vi "Create.vi"() -> (8 "Moving Ripple Noise":refnum<class "Moving Ripple Noise.lvclass">)   [LabVIEW 2020, in "Moving Ripple Noise.lvclass"]
uses:
  Moving Ripple Noise.lvclass
  Moving Ripple Noise.lvclass/Moving Ripple Noise.ctl
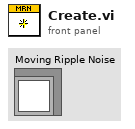
[diagram p1: front panel]
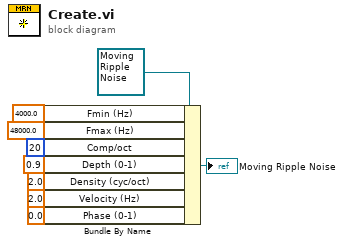
[diagram p0: block diagram]
diagram:
  n1 = Bundle By Name(cluster=refnum<class "Moving Ripple Noise.lvclass"> refnum ("Moving Ripple Noise"), "Fmin (Hz)"=4000.0 ("Serialized.Fmin"), "Fmax (Hz)"=48000.0 ("Serialized.Fmax"), "Comp/oct"=20 ("Serialized.Comp/oct"), "Depth (0-1)"=0.9 ("Serialized.Depth"), "Density (cyc/oct)"=2.0 ("Serialized.Density"), "Velocity (Hz)"=2.0 ("Serialized.Velocity"), "Phase (0-1)"=0.0 ("Serialized.Phase")) -> (→"Moving Ripple Noise":refnum<class "Moving Ripple Noise.lvclass">)
